vi "AddSubscriber.vi"(8 "ErrorIn":errorcluster, 9 "Filters":T1[](array[typedef]), 11 "ITAFFilteredTrace in":refnum<class "ITAFFilteredTrace.lvclass">) -> (0 "ErrorOut":errorcluster, 1 "TraceQueue":refnum<queue>, 3 "ITAFFilteredTrace out":refnum<class "ITAFFilteredTrace.lvclass">)   [LabVIEW 2021, in "ITAFFilteredTrace.lvclass"]
uses:
  ITAFFilteredTrace.lvclass
  Library_TAF_TraceWindow/TAFTraceWindow/FilterConfiguration.ctl
  Library_TAF_TraceWindow/TAFTraceWindow/FilterFunction.ctl
  Library_TAF_TraceWindow/TAFTraceWindow/TAFTraceWindow.lvclass
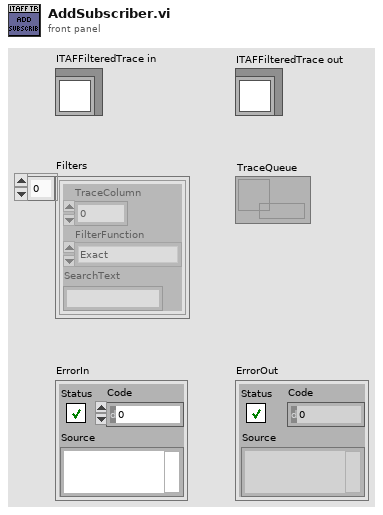
[diagram p1: front panel]
types:
  T1 = typedef "TAFTraceWindow.lvclass/FilterConfiguration.ctl" = cluster{"TraceColumn":i32, "FilterFunction":T2, "SearchText":string}
  T2 = typedef "TAFTraceWindow.lvclass/FilterFunction.ctl" = enum16{"Exact", "Regex"}
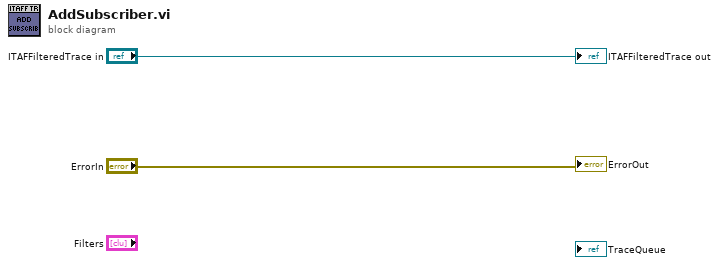
[diagram p0: block diagram]
diagram:
  "ErrorOut" <- "ErrorIn"
  "ITAFFilteredTrace out" <- "ITAFFilteredTrace in"
